vi "getTRMregs.vi"(11 "VISA Refnum in":refnum<visa-resource-name>) -> (0 "error out":errorcluster, 1 "Setpoint":i16, 2 "Temp":i16)   [LabVIEW 2020]
uses:
  <vilib>/NI Modbus.llb/MB Serial Master Query Read Holding Registers (poly).vi
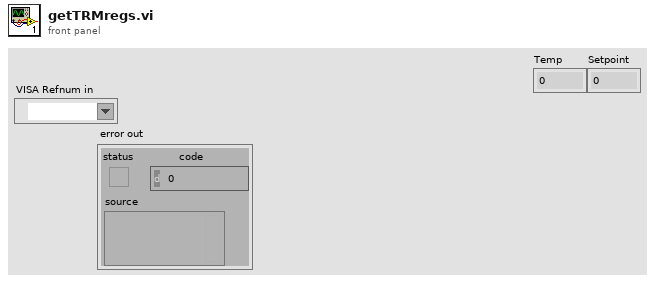
[diagram p1: front panel]
types:
  T1 = cluster{"Mode":enum16{"RTU", "ASCII"}, "Slave Address":u8}
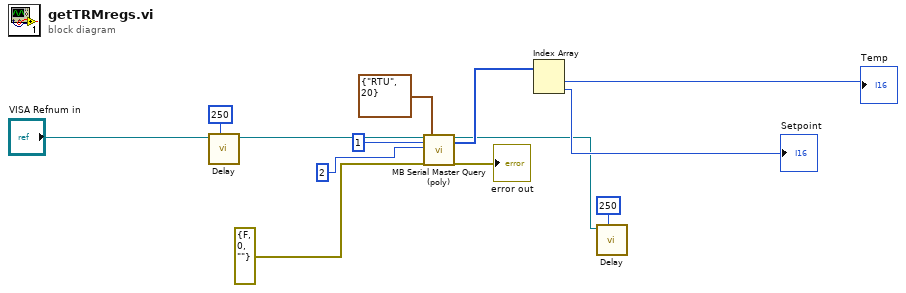
[diagram p0: block diagram]
diagram:
  n1 = call "Delay.vi"("milliseconds to wait"=u32 250, "VISA Refnum  In"="VISA Refnum in") -> ("VISA Refnum out"=w4:refnum<visa-resource-name>)  [unwired: 8 in, 1 out]
  n2 = call-poly <vilib>:"MB Serial Master Query (poly).vi"("VISA resource name"=w4, "Starting Address"=u16 1, "Quantity"=u16 2, "error in"=errorcluster {"status"=FALSE, "code"=0, "source"=""} ("error out"), "Serial Parameters"=T1 {"Mode"=enum."RTU", "Slave Address"=20}) -> ("VISA resource name out"=w2:refnum<visa-resource-name>, "Holding Registers"=w9:u16[], "error out"=→"error out":errorcluster)  [unwired: 1 in, 11 out]
  n3 = Index Array(array=w9) -> (element #1=→"Temp":u16, element #2=→"Setpoint":u16)  [unwired: 2 in]
  n4 = call "Delay.vi"("milliseconds to wait"=u32 250, "VISA Refnum  In"=w2) -> ()  [unwired: 8 in, 2 out]
